vi "call_python_node.vi"() -> ()   [LabVIEW 2019]
panel:
  in  "module relative path":string
  out "error out":errorcluster
  in  "error in (no error)":errorcluster
  in  "function name":string
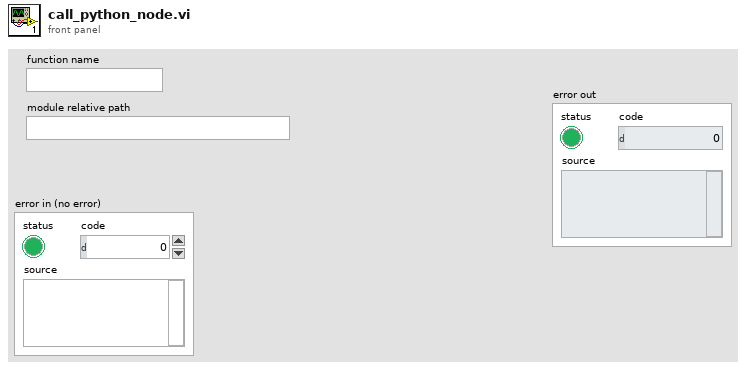
[diagram p1: front panel]
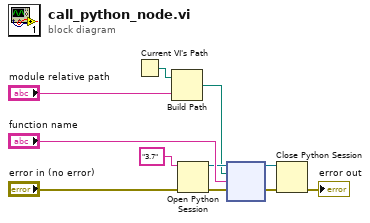
[diagram p0: block diagram]
diagram:
  n1 = Current VI's Path() -> (path=w3:path)
  n2 = Build Path(base path=w3, name or relative path="module relative path") -> (appended path=w1:path)
  n3 = Open Python Session(python version="3.7" ("Python version"), 3:"error in (no error)") -> (session out=w4:refnum<k35>, error out=w7:errorcluster)  [unwired: 1 in]
  n4 = node(w4, w1, "function name", w7) -> (w10:refnum<k35>, w9:errorcluster)  [unwired: 2 in, 2 out]
  n5 = Close Python Session(session in=w10, error in=w9) -> (11:→"error out":errorcluster)
